vi "Execute.vi"(8 "error in (no error)":errorcluster, 9 "Consumer Queues in":T1, 10 "UI Process Command in":refnum<class "UI Idle State.lvclass">, 11 "UI Process Data in":T2) -> (0 "error out":errorcluster, 1 "Consumer Queues out":T1, 2 "Stop?":bool, 3 "UI Process Data out":T2)   [LabVIEW 2019, in "User Interface Process.lvlib" / "UI Idle State.lvclass"]
uses:
  UI Idle State.lvclass
  C:/Users/wg/Documents/LV_Projects/TestStand/App/UI Process/Generic UI Command/Generic UI Process Command.lvclass
  UI Process Data.ctl
  TS Framework/ExeLogging/UI Logger/UI Logger.lvclass
  UI State.ctl
  TS Framework/Consumer Queues.ctl
  Generic UI Command/Generic UI Process Command.lvclass
  DAC Process/Generic DAC Command/Generic DAC Process Command.lvclass
  Trig Process/Generic Trig Command/Generic Trig Process Command.lvclass
  User Interface Process.lvlib
  TS Framework/TS Framework.lvlib
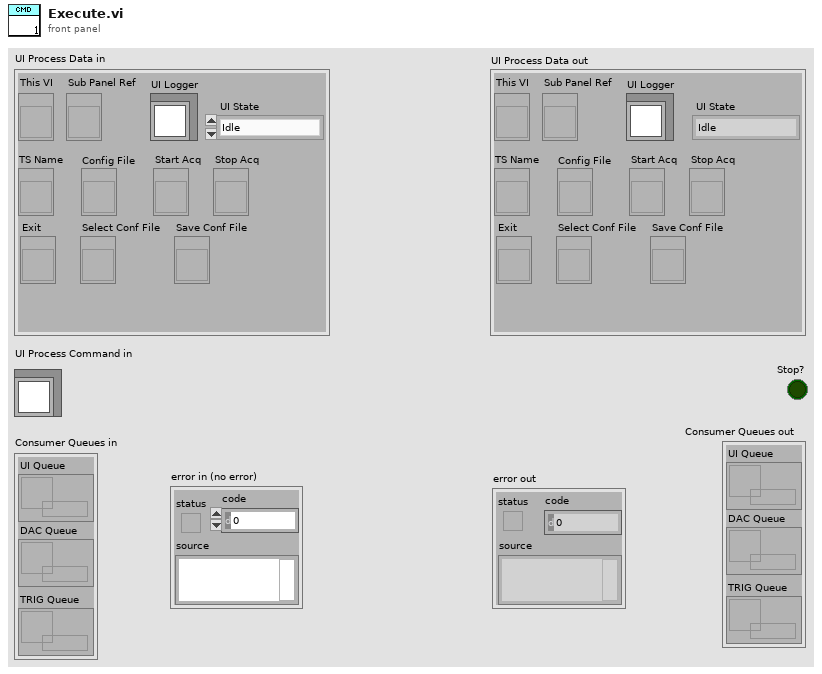
[diagram p1: front panel]
types:
  T1 = typedef "TS Framework.lvlib/Consumer Queues.ctl" = cluster{"UI Queue":refnum<queue>, "DAC Queue":refnum<queue>, "TRIG Queue":refnum<queue>}
  T2 = typedef "User Interface Process.lvlib/UI Process Data.ctl" = cluster{"This VI":refnum<vi>, "Sub Panel Ref":refnum<vi>, "UI Logger":refnum<class "UI Logger.lvclass">, "TS Name":refnum<vi>, "Config File":refnum<vi>, "Start Acq":refnum<vi>, "Stop Acq":refnum<vi>, "Exit":refnum<vi>, "Select Conf File":refnum<vi>, "Save Conf File":refnum<vi>, "UI State":T3}
  T3 = typedef "User Interface Process.lvlib/UI State.ctl" = enum16{"Idle", "Acquiring"}
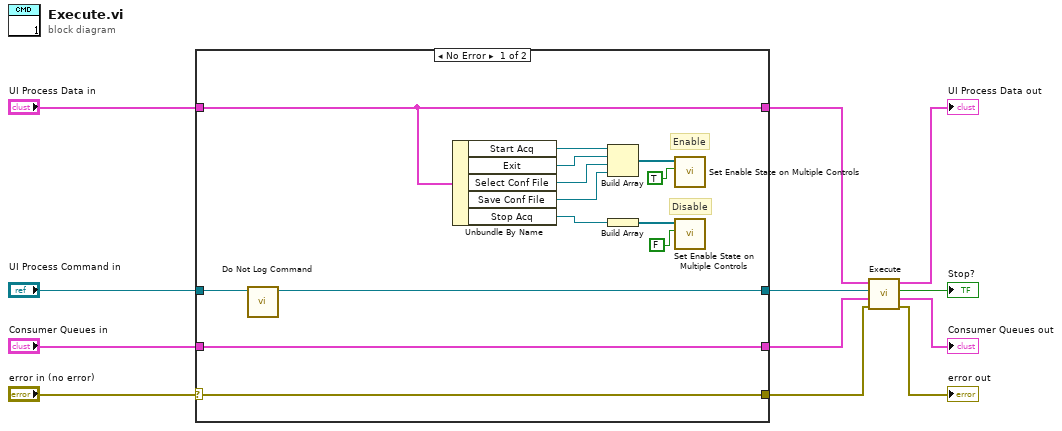
[diagram p0: block diagram]
diagram:
  n1 = case shown="No Error" "error in (no error)" {
    selector: "error in (no error)" -> [w14 w27]
    tunnel: "UI Process Command in" -> [w26 w30]
    tunnel: "UI Process Data in" -> [w15 w29]
    tunnel: [w25 w30] -> w4
    tunnel: [w15 w29] -> w1
    tunnel: "Consumer Queues in" -> [w24 w28]
    tunnel: [w24 w28] -> w3
    tunnel: [w14 w27] -> w2
    frame No Error {
      # "Enable"
      # "Disable"
      n2 = call "Do Not Log Command.vi"("UI Process Command in"=w26) -> ("UI Process Command out"=w25:refnum<class "UI Idle State.lvclass">)  [unwired: 10 in]
      n3 = Unbundle By Name(w15) -> ("Start Acq"=w16:refnum<vi>, "Exit"=w17:refnum<vi>, "Select Conf File"=w19:refnum<vi>, "Save Conf File"=w18:refnum<vi>, "Stop Acq"=w13:refnum<vi>)
      n4 = Build Array(w16, w17, w19, w18) -> (w20:refnum<vi>[])
      n5 = Build Array(w13) -> (w21:refnum<vi>[])
      n6 = call "Set Enable State on Multiple Controls.vi"("Enable?"=TRUE, "Controls"=w20) -> ()  [unwired: 10 in]
      n7 = call "Set Enable State on Multiple Controls.vi"("Enable?"=FALSE, "Controls"=w21) -> ()  [unwired: 10 in]
    }
    frame Error {
    }
  }
  n8 = call-parent "Execute.vi"("error in (no error)"=w2, "Consumer Queues in"=w3, "UI Process Command in"=w4, "UI Process Data in"=w1) -> ("error out"=→"error out":errorcluster, "Consumer Queues out"=→"Consumer Queues out":T1, "Stop?"=→"Stop?":bool, "UI Process Data out"=→"UI Process Data out":T2)  [unwired: 4 in]
